vi "getSerializedData.vi"(0 "reference":refnum<class "InterfaceNode.lvclass">, 5 "error in (no error)":errorcluster) -> (14 "reference out":refnum<class "InterfaceNode.lvclass">, 15 "parent":refnum<class "AbstractNode.lvclass">, 16 "children":refnum<class "AbstractNode.lvclass">[](array[class]), 17 "xmlOut":string, 19 "error out":errorcluster)   [LabVIEW 2016, in "InterfaceNode.lvclass"]
doc: "getSerializedData"
uses:
  <resource>/Framework/Providers/Open_GDS/UML/InterfaceNode_class/InterfaceNode.lvclass
  C:/Program Files (x86)/National Instruments/LabVIEW 2016/resource/Framework/Providers/Open_GDS/UML/RectangularNode_class/RectangularNode.lvclass
  C:/Program Files (x86)/National Instruments/LabVIEW 2016/resource/Framework/Providers/Open_GDS/UML/AbstractNode_class/AbstractNode.lvclass
  <resource>/Framework/Providers/Open_GDS/UML/AbstractNode_class/AbstractNode.lvclass
  <resource>/Framework/Providers/Open_GDS/UML/General/Rectangle/Rectangle Rectangle2D.ctl
  <resource>/Framework/Providers/Open_GDS/UML/MultiLineString_class/MultiLineString.lvclass
  <resource>/Framework/Providers/Open_GDS/UML/RectangularNode_class/RectangularNode.lvclass
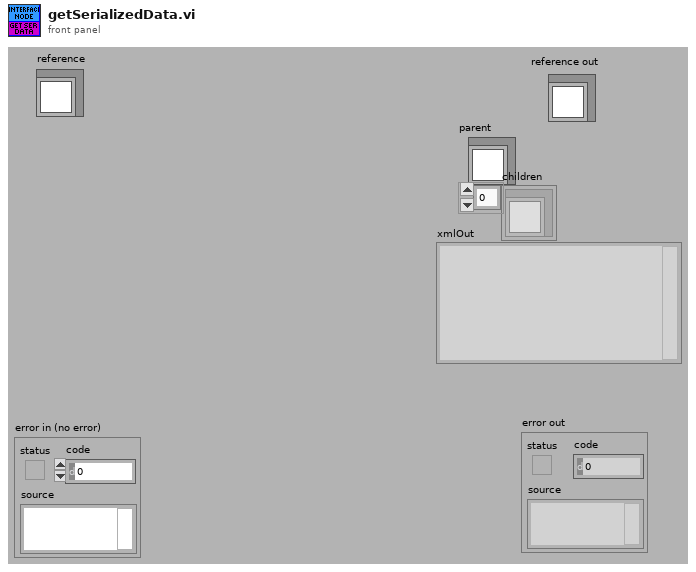
[diagram p1: front panel]
types:
  T1 = typedef "Rectangle Rectangle2D.ctl" = cluster{"x":dbl, "y":dbl, "width":dbl, "height":dbl}
  T2 = cluster{"Base class":cluster{"Base class":cluster{"parent":refnum<k1>, "children":refnum<k1>[], "Hidden":bool}, "bounds":T1}, "midHeight":dbl, "botHeight":dbl, "name":refnum<k1>, "methods":refnum<k1>, "DEFAULT_COMPARTMENT_HEIGHT":i32, "DEFAULT_WIDTH":i32, "DEFAULT_HEIGHT":i32}
  T3 = typedef "InterfaceNode.lvclass/ObjectAttributes.ctl" = cluster{"midHeight":dbl, "botHeight":dbl, "name":refnum<class "MultiLineString.lvclass">, "methods":refnum<class "MultiLineString.lvclass">, "DEFAULT_COMPARTMENT_HEIGHT":i32, "DEFAULT_WIDTH":i32, "DEFAULT_HEIGHT":i32}
  T4 = typedef "RectangularNode.lvclass/ObjectAttributes.ctl" = cluster{"bounds":T1}
  T5 = typedef "AbstractNode.lvclass/ObjectAttributes.ctl" = cluster{"parent":refnum<class "AbstractNode.lvclass">, "children":refnum<class "AbstractNode.lvclass">[], "Hidden":bool}
  T6 = cluster{"Attributes":cluster{"Base class":cluster{"Base class":cluster{"parent":refnum<k1>, "children":refnum<k1>[], "Hidden":bool}, "bounds":T1}, "midHeight":dbl, "botHeight":dbl, "name":refnum<k1>, "methods":refnum<k1>, "DEFAULT_COMPARTMENT_HEIGHT":i32, "DEFAULT_WIDTH":i32, "DEFAULT_HEIGHT":i32}, "text":string, "text":string}
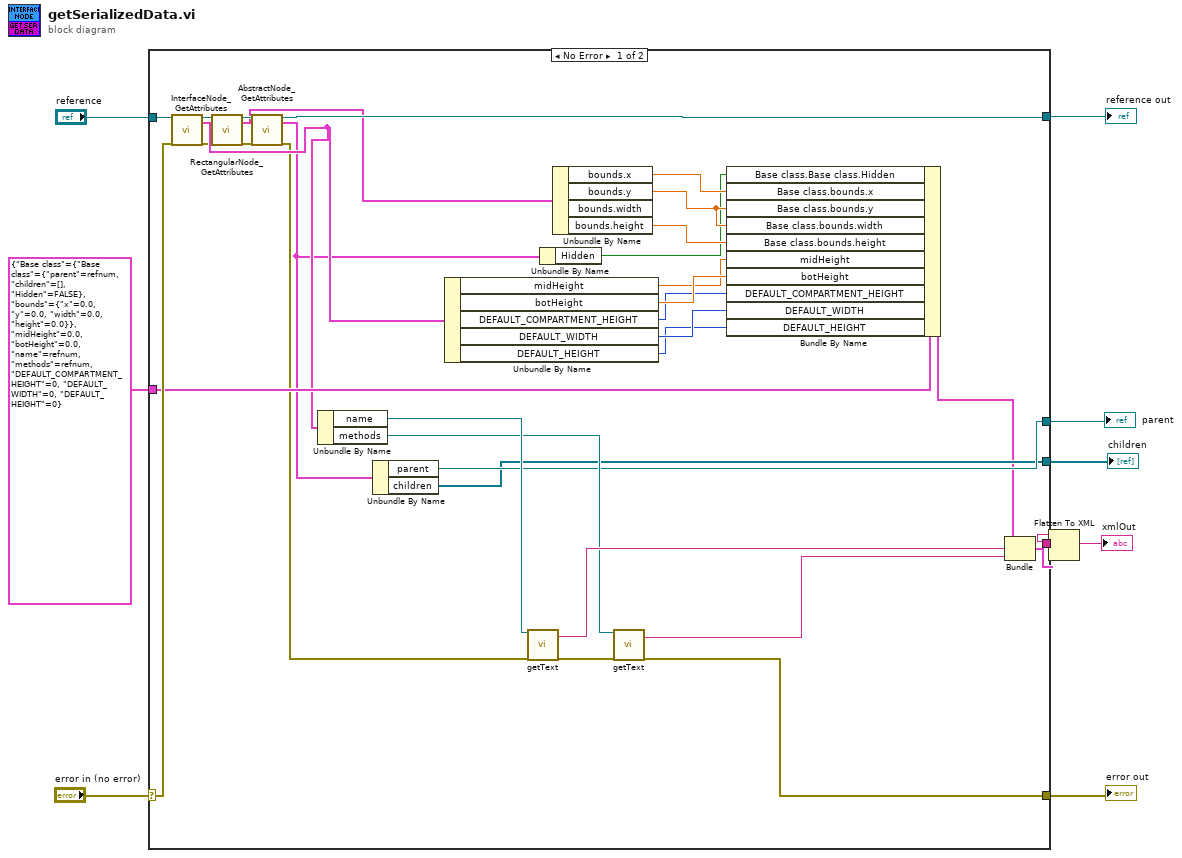
[diagram p0: block diagram]
diagram:
  n1 = case shown="No Error" "error in (no error)" {
    selector: "error in (no error)" -> [w40 w41]
    tunnel: "reference" -> [w39 w42]
    tunnel: [w32 w41] -> w6
    tunnel: [w11 w42] -> w5
    tunnel: [w31 _] -> w4
    tunnel: [w30 _] -> w3
    tunnel: [w29 _] -> w2
    tunnel: T2 {"Base class"={"Base class"={"parent"=refnum, "children"=[], "Hidden"=FALSE}, "bounds"={"x"=0.0, "y"=0.0, "width"=0.0, "height"=0.0}}, "midHeight"=0.0, "botHeight"=0.0, "name"=refnum, "methods"=refnum, "DEFAULT_COMPARTMENT_HEIGHT"=0, "DEFAULT_WIDTH"=0, "DEFAULT_HEIGHT"=0} ("Attributes") -> [w20 _]
    frame No Error {
      n2 = call <resource>:"InterfaceNode_GetAttributes.vi"("reference in"=w39, "error in (no error)"=w40) -> ("reference out"=w16:refnum<class "InterfaceNode.lvclass">, "Data"=w17:T3, "error out"=w15:errorcluster)  [unwired: 1 in, 14 out]
      n3 = call <resource>:"RectangularNode_GetAttributes.vi"("reference in"=w16, "error in (no error)"=w15) -> ("reference out"=w14:refnum<class "InterfaceNode.lvclass">, "Data"=w9:T4, "error out"=w13:errorcluster)  [unwired: 14 in, 1 out]
      n4 = call <resource>:"AbstractNode_GetAttributes.vi"("reference in"=w14, "error in (no error)"=w13) -> ("reference out"=w11:refnum<class "InterfaceNode.lvclass">, "Data"=w10:T5, "error out"=w12:errorcluster)  [unwired: 14 in, 1 out]
      n5 = Unbundle By Name(w17) -> ("name"=w37:refnum<class "MultiLineString.lvclass">, "methods"=w34:refnum<class "MultiLineString.lvclass">)
      n6 = Unbundle By Name(w10) -> ("parent"=w31:refnum<class "AbstractNode.lvclass">, "children"=w30:refnum<class "AbstractNode.lvclass">[])
      n7 = Unbundle By Name(w17) -> ("midHeight"=w24:dbl, "botHeight"=w25:dbl, "DEFAULT_COMPARTMENT_HEIGHT"=w23:i32, "DEFAULT_WIDTH"=w22:i32, "DEFAULT_HEIGHT"=w21:i32)
      n8 = call-dynamic "getText.vi"("reference"=w37, "error in (no error)"=w12) -> ("text"=w36:string, "error out"=w33:errorcluster)  [unwired: 16 out]
      n9 = Unbundle By Name(w10) -> ("Hidden"=w18:bool)
      n10 = Unbundle By Name(w9) -> ("bounds.x"=w28:dbl, "bounds.y"=w27:dbl, "bounds.height"=w26:dbl)  [unwired: 1 out]
      n11 = call-dynamic "getText.vi"("reference"=w34, "error in (no error)"=w33) -> ("text"=w35:string, "error out"=w32:errorcluster)  [unwired: 16 out]
      n12 = Bundle By Name(cluster=w20, "Base class.Base class.Hidden"=w18, "Base class.bounds.x"=w28, "Base class.bounds.y"=w27, "Base class.bounds.width"=w27, "Base class.bounds.height"=w26, "midHeight"=w24, "botHeight"=w25, "DEFAULT_COMPARTMENT_HEIGHT"=w23, "DEFAULT_WIDTH"=w22, "DEFAULT_HEIGHT"=w21) -> (w19:T2)
      n13 = Bundle("Attributes"=w19, "text"=w36, "text"=w35) -> (w38:T6)  [unwired: 1 out]
      n14 = Flatten To XML(anything=w38) -> (xml string=w29:string)
    }
    frame Error {
    }
  }
  "reference out" <- w5
  "error out" <- w6
  "parent" <- w4
  "children" <- w3
  "xmlOut" <- w2
